vi "EditorSub dataToListbox.vi"(7 "currFilePath":path, 8 "error in (no error)":errorcluster, 10 "listboxColHead":string[](array[string])=["Index", "Name", "Plot", "M/Z", "Intensity", "Center Point", "Left Point", "Right Point", "Half Height", "Remark"], 11 "newSigInfo in":T1={"startTime"=0.0, "scanData"=[], "xyXLabel"="m/z (Th)", "xyYLabel"="Intensity (V)", "peakData"=[]}) -> (0 "error out":errorcluster, 3 "newSigInfo out":T1={"startTime"=0.0, "scanData"=[], "xyXLabel"="m/z (Th)", "xyYLabel"="Intensity (V)", "peakData"=[]}, 5 "Item Names":string[][](array[string]))   [LabVIEW 2018]
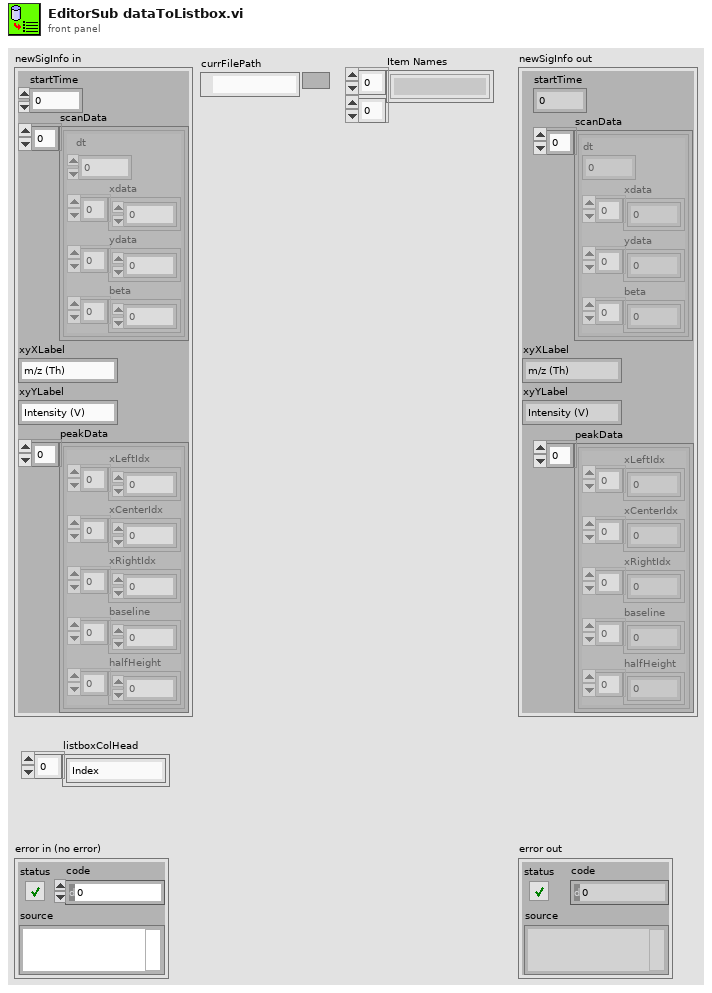
[diagram p1: front panel]
types:
  T1 = cluster{"startTime":dbl, "scanData":cluster{"dt":dbl, "xdata":dbl[], "ydata":sgl[], "beta":dbl[]}[], "xyXLabel":string, "xyYLabel":string, "peakData":cluster{"xLeftIdx":u32[], "xCenterIdx":u32[], "xRightIdx":u32[], "baseline":sgl[], "halfHeight":dbl[]}[]}
  T2 = cluster{"dt":dbl, "xdata":dbl[], "ydata":sgl[], "beta":dbl[]}[]
  T3 = cluster{"xLeftIdx":u32[], "xCenterIdx":u32[], "xRightIdx":u32[], "baseline":sgl[], "halfHeight":dbl[]}[]
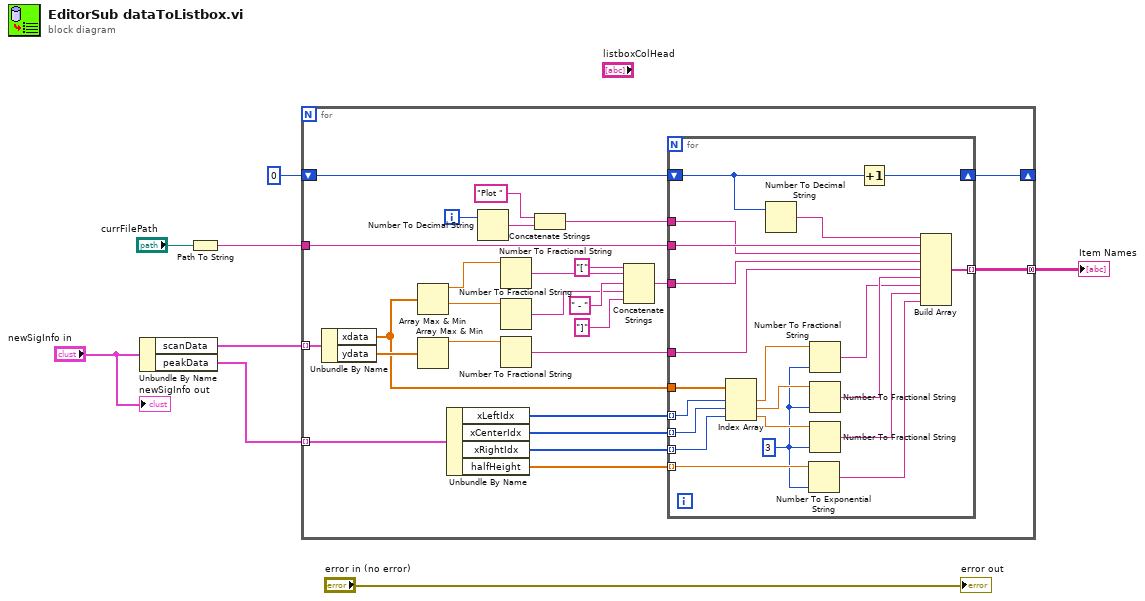
[diagram p0: block diagram]
diagram:
  n1 = Unbundle By Name("newSigInfo in") -> ("scanData"=w8:T2, "peakData"=w7:T3)
  n2 = Path To String(path="currFilePath") -> (string=w5:string)
  n3 = for {
    tunnel: w8 -> [w32] mode=indexing
    tunnel: w7 -> [w33] mode=indexing
    tunnel: w5 -> [w34]
    shift-right: [w30] -> _
    shift-left: 0 -> [w31]
    tunnel: [w10] -> w3 mode=concatenating
    i -> [w28]
    n4 = Unbundle By Name(w32) -> ("xdata"=w9:dbl[], "ydata"=w29:sgl[])
    n5 = Array Max & Min(array=w9) -> (max value=w24:dbl, min value=w23:dbl)  [unwired: 2 out]
    n6 = Array Max & Min(array=w29) -> (max value=w22:sgl)  [unwired: 3 out]
    n7 = Unbundle By Name(w33) -> ("xLeftIdx"=w14:u32[], "xCenterIdx"=w13:u32[], "xRightIdx"=w12:u32[], "halfHeight"=w11:dbl[])
    n8 = Number To Decimal String(number=w28) -> (decimal integer string=w26:string)  [unwired: 1 in]
    n9 = Number To Fractional String(number=w24) -> (F-format string=w20:string)  [unwired: 3 in]
    n10 = Number To Fractional String(number=w23) -> (F-format string=w18:string)  [unwired: 3 in]
    n11 = Number To Fractional String(number=w22) -> (F-format string=w15:string)  [unwired: 3 in]
    n12 = Concatenate Strings("Plot ", w26) -> (w25:string)
    n13 = Concatenate Strings("[", w20, " - ", w18, "]") -> (w16:string)
    n14 = for {
      tunnel: w34 -> [w55]
      shift-right: [w54] -> w30
      shift-left: w31 -> [w53]
      tunnel: w25 -> [w51]
      tunnel: w16 -> [w50]
      tunnel: w15 -> [w49]
      tunnel: w14 -> [w41] mode=indexing
      tunnel: w13 -> [w40] mode=indexing
      tunnel: w12 -> [w39] mode=indexing
      tunnel: w11 -> [w48] mode=indexing
      tunnel: [w43] -> w10 mode=indexing
      tunnel: w9 -> [w42]
      w35 = i16 3 ("precision (6)")
      n15 = Index Array(array=w42, index #1=w41, index #2=w40, index #3=w39) -> (element #1=w38:dbl, element #2=w37:dbl, element #3=w36:dbl)
      n16 = Number To Decimal String(number=w53) -> (decimal integer string=w52:string)  [unwired: 1 in]
      n17 = Number To Exponential String(number=w48, precision (6)=w35) -> (E-format string=w44:string)  [unwired: 2 in]
      n18 = Number To Fractional String(number=w38, precision (6)=w35) -> (F-format string=w46:string)  [unwired: 2 in]
      n19 = Number To Fractional String(number=w37, precision (6)=w35) -> (F-format string=w47:string)  [unwired: 2 in]
      n20 = Number To Fractional String(number=w36, precision (6)=w35) -> (F-format string=w45:string)  [unwired: 2 in]
      n21 = Increment(x=w53) -> (x+1=w54:i32)
      n22 = Build Array(w52, w55, w51, w50, w49, w47, w46, w45, w44) -> (w43:string[])
    }
  }
  "Item Names" <- w3
  "error out" <- "error in (no error)"
  "newSigInfo out" <- "newSigInfo in"
